vi "Order Analysis Functions Demo.vi"() -> ()   [LabVIEW 2017]
doc: "This the VI that shows all toolkit features."
panel:
  out "left_top":bool
  out "status":string
  out "selected item":string
  in  "STOP":bool
  in  "tree":string(tree)="Toolkit Features"
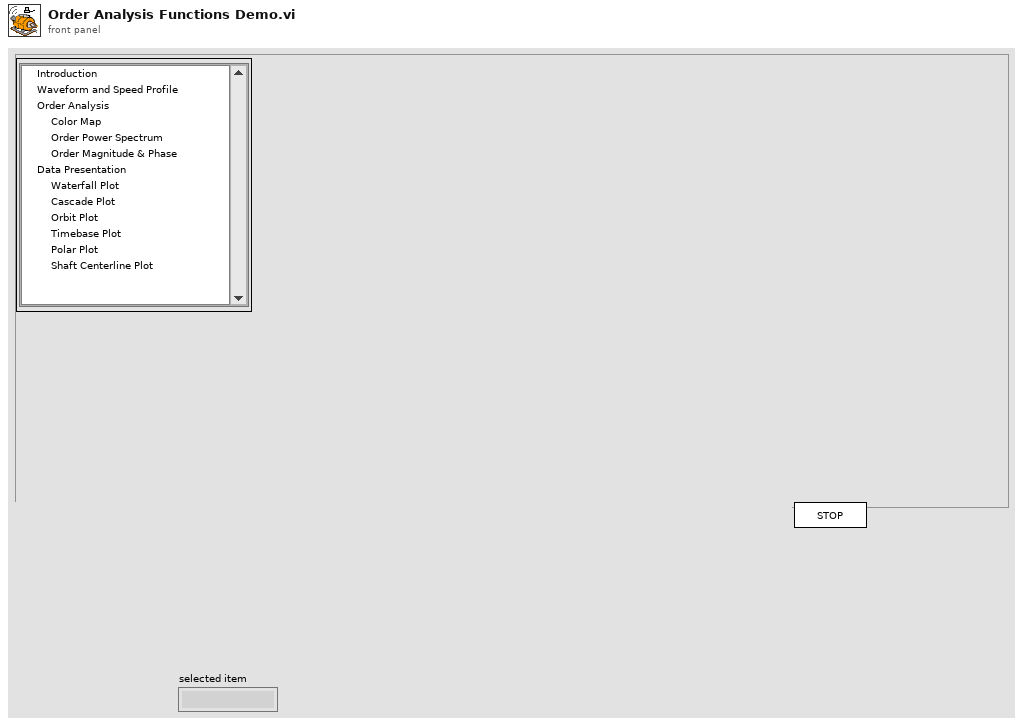
[diagram p1: front panel]
types:
  T1 = typedef "LVPositionTypeDef.ctl" = cluster{"Left":i32, "Top":i32}
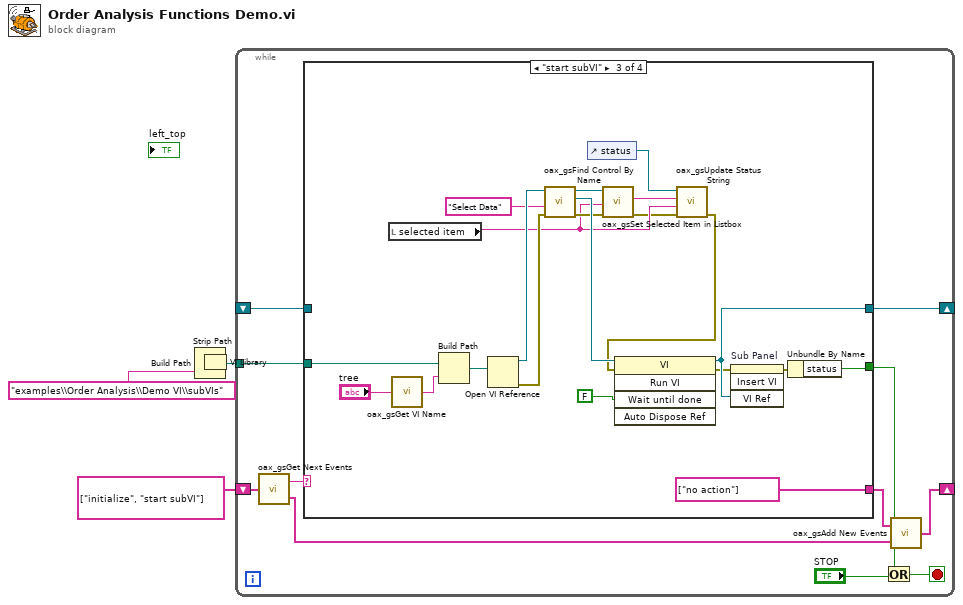
[diagram p0: block diagram]
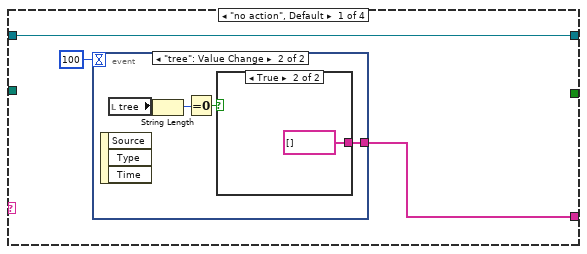
[diagram p2: hidden frame]
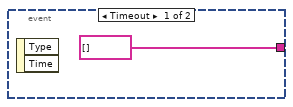
[diagram p3: hidden frame]
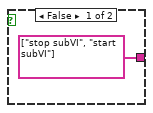
[diagram p4: hidden frame]
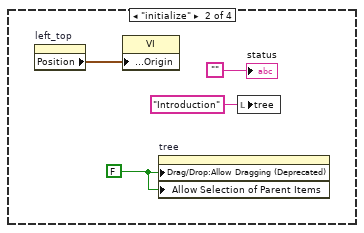
[diagram p5: hidden frame]
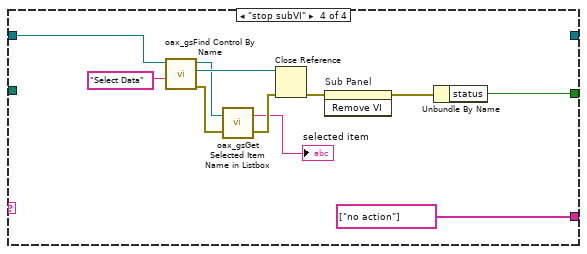
[diagram p6: hidden frame]
diagram:
  n1 = VI Library() -> (path=w4:path)
  n2 = Strip Path(path=w4) -> (stripped path=w5:path)  [unwired: 1 out]
  n3 = Build Path(base path=w5, name or relative path="examples\\Order Analysis\\Demo VI\\subVIs") -> (appended path=w2:path)
  n4 = while {
    tunnel: w2 -> [w16]
    shift-right: [w15] -> _
    shift-left: _ -> [w14]
    shift-right: [w9] -> _
    shift-left: string[] ["initialize", "start subVI"] -> [w13]
    stop <- w6 stop-if-true
    n5 = call <vilib>:"oax_gsGet Next Events.vi"("event queue in"=w13) -> ("next event"=w12:string, "event queue out"=w11:string[])
    n6 = case shown="\"start subVI\"" w12 {
      tunnel: w16 -> [_ _ w51 _]
      tunnel: [w19 _ w49 _] -> w15
      tunnel: w14 -> [w19 _ _ w58]
      tunnel: [_ _ w50 w62] -> w7
      tunnel: [w17 _ string[] ["no action"] string[] ["no action"]] -> w10
      frame "no action", Default {
        n7 = event shown="[1] \"tree\": Value Change" {
          selector: _ -> [_ _]
          dyn-events: _ -> [_ _]
          timeout: 100 -> [_ _]
          tunnel: [string[] [] ("f") w24] -> w17
          event Timeout {
            n8 = event-data() -> ()  [unwired: 1 in, 2 out]
          }
          event "tree": Value Change {
            n9 = event-data() -> ()  [unwired: 1 in, 3 out]
            n10 = local read "tree"() -> (w22:string)
            n11 = String Length(string=w22) -> (length=w23:i32)
            n12 = Equal To 0?(x=w23) -> (x = 0?=w21:bool)
            n13 = case shown="True" w21 {
              tunnel: [string[] ["stop subVI", "start subVI"] string[] []] -> w24
              frame False {
              }
              frame True {
              }
            }
          }
        }
      }
      frame "initialize" {
        w28 = FALSE ("Allow Dragging")
        n14 = property on="left_top" class="Bool (strict)"() -> ("Position"=w27:T1)  [unwired: 2 in, 2 out]
        n15 = property class="VI"("Front Panel Window:Origin"=w27) -> ()  [unwired: 2 in, 2 out]
        n16 = property on="tree" class="Tree (strict)"("Drag/Drop:Allow Dragging (Deprecated)"=w28, "Allow Selection of Parent Items"=w28) -> ()  [unwired: 2 in, 2 out]
        n17 = local write "tree"("Introduction" ("tree")) -> ()
        "status" <- ""
      }
      frame "start subVI" {
        n18 = local read "selected item"() -> (w34:string)
        n19 = call <vilib>:"oax_gsGet VI Name.vi"("tree"="tree") -> ("vi name"=w46:string)
        n20 = Build Path(base path=w51, name or relative path=w46) -> (appended path=w45:path)
        n21 = Open VI Reference(vi path=w45) -> (vi reference=w40:refnum<vi>, error out=w41:errorcluster)  [unwired: 5 in]
        n22 = call <vilib>:"oax_gsFind Control By Name.vi"("error in (no error)"=w41, "control name"="Select Data", "vi refnum in"=w40) -> ("error out"=w36:errorcluster, "vi refnum out"=w39:refnum<vi>, "control refnum"=w37:refnum<vi>)  [unwired: 6 in]
        n23 = control-ref of="status"() -> (w35:refnum<vi>)
        n24 = call <vilib>:"oax_gsSet Selected Item in Listbox.vi"("error in (no error)"=w36, "item name"=w34, "control refnum"=w37) -> ("error out"=w32:errorcluster, "actual item name"=w33:string)  [unwired: 6 in, 1 out]
        n25 = call <vilib>:"oax_gsUpdate Status String.vi"("error in (no error)"=w32, "old status"=w34, "new status"=w33, "Ctl Refnum"=w35) -> ("error out"=w31:errorcluster)  [unwired: 3 in]
        n26 = invoke class="VI" method="Run VI"(reference=w39, error in=w31, "Wait until done"=FALSE) -> (reference out=w49:refnum<vi>, error out=w43:errorcluster)  [unwired: 2 in, 3 out]
        n27 = invoke on="Sub Panel" class="SubPanel" method="Insert VI"(error in=w43, "VI Ref"=w49) -> (error out=w42:errorcluster)  [unwired: 2 in, 3 out]
        n28 = Unbundle By Name(w42) -> ("status"=w50:bool)
      }
      frame "stop subVI" {
        n29 = call <vilib>:"oax_gsFind Control By Name.vi"("control name"="Select Data", "vi refnum in"=w58) -> ("error out"=w54:errorcluster, "vi refnum out"=w57:refnum<vi>, "control refnum"=w55:refnum<vi>)  [unwired: 7 in]
        n30 = call <vilib>:"oax_gsGet Selected Item Name in Listbox.vi"("error in (no error)"=w54, "ctrl reference"=w55) -> ("error out"=w53:errorcluster, "selected item"=→"selected item":string)
        n31 = Close Reference(reference=w57, error in (no error)=w53) -> (error out=w60:errorcluster)
        n32 = invoke on="Sub Panel" class="SubPanel" method="Remove VI"(error in=w60) -> (error out=w59:errorcluster)  [unwired: 2 in, 2 out]
        n33 = Unbundle By Name(w59) -> ("status"=w62:bool)
      }
    }
    n34 = Or(x=w7, y="STOP") -> (x .or. y?=w6:bool)
    n35 = call <vilib>:"oax_gsAdd New Events.vi"("event in"=w11, "new events"=w10) -> ("event out"=w9:string[])
  }
